vi "csvSim.vi"() -> ()   [LabVIEW 2021]
uses:
  <vilib>/Utility/file.llb/Write Delimited Spreadsheet (string).vi
  <vilib>/Utility/file.llb/Write Delimited Spreadsheet (DBL).vi
panel:
  in  "Path":path
  in  "stop":bool
  in  "Channel":string[](array[string])
  in  "Header information":string[][](array[string])
  in  "Number to write":i16
  in  "Number of channels":u8
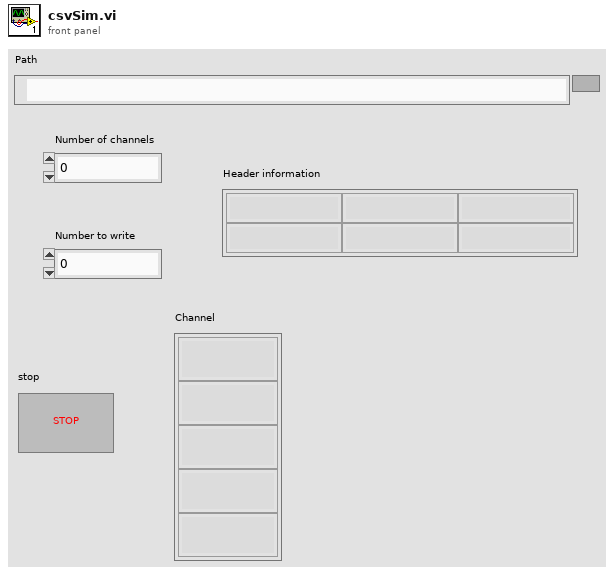
[diagram p1: front panel]
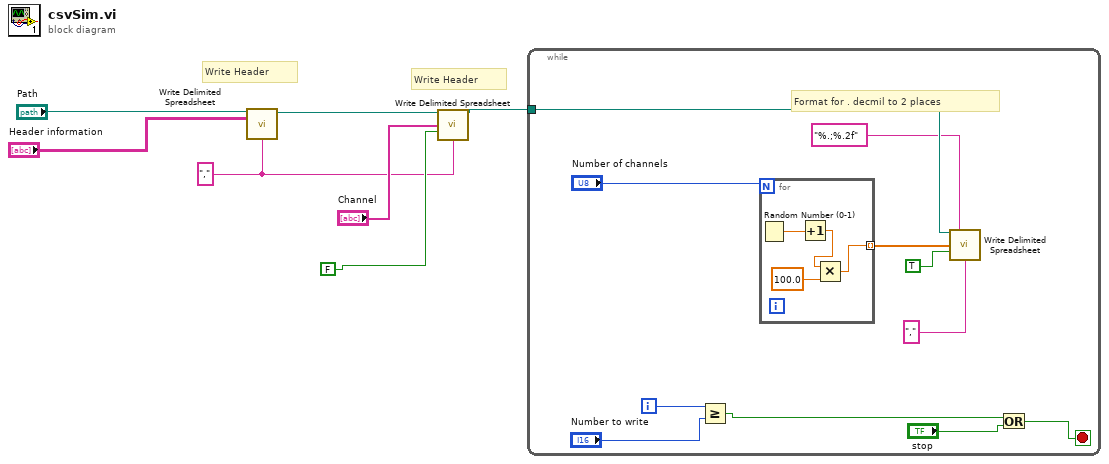
[diagram p0: block diagram]
diagram:
  w2 = "," ("delimiter (\\t)")
  # "Write Header"
  # "Write Header"
  n1 = call-poly <vilib>:"Write Delimited Spreadsheet.vi"("file path (dialog if empty)"="Path", "2D data"="Header information", "delimiter (\\t)"=w2) -> ("new file path (Not A Path if cancelled)"=w5:path)  [unwired: 11 in, 1 out]
  n2 = call-poly <vilib>:"Write Delimited Spreadsheet.vi"("file path (dialog if empty)"=w5, "1D data"="Channel", "append to file? (new file:F)"=FALSE, "delimiter (\\t)"=w2) -> ("new file path (Not A Path if cancelled)"=w1:path)  [unwired: 10 in, 1 out]
  n3 = while {
    tunnel: w1 -> [w12]
    i -> [w15]
    stop <- w17 stop-if-true
    # "Format for . decmil to 2 places"
    n4 = Greater Or Equal?(x=w15, y="Number to write") -> (x >= y?=w14:bool)
    n5 = for {
      N: "Number of channels" -> [_]
      tunnel: [w22] -> w11 mode=indexing
      n6 = Random Number (0-1)() -> (number: 0 to 1=w20:dbl)
      n7 = Increment(x=w20) -> (x+1=w19:dbl)
      n8 = Multiply(x=w19, y=100.0) -> (x*y=w22:dbl)
    }
    n9 = call-poly <vilib>:"Write Delimited Spreadsheet.vi"("file path (dialog if empty)"=w12, "format (%.3f)"="%.;%.2f", "1D data"=w11, "append to file? (new file:F)"=TRUE, "delimiter (\\t)"="," ("delimiter (\\t)")) -> ()  [unwired: 9 in, 2 out]
    n10 = Or(x=w14, y="stop") -> (x .or. y?=w17:bool)
  }
